vi "HTML.vi"() -> ()   [LabVIEW 2013]
uses:
  <vilib>/Utility/NIReport.llb/NI_report.lvclass
  <vilib>/Utility/NIReport.llb/Append Report Text (str wrap).vi
  <vilib>/Utility/NIReport.llb/Append Text Table to Report (wrap).vi
  <vilib>/Utility/NIReport.llb/Append Image to Report (path wrap).vi
  <vilib>/printing/OpenHTMLReport.llb/Open HTML Report in Browser (Refnum).vi
  <vilib>/Utility/NIReport.llb/NI_ReportGenerationCore.lvlib
panel:
  in  "list elements":string[](array[string])
  in  "column headers":string[](array[string])
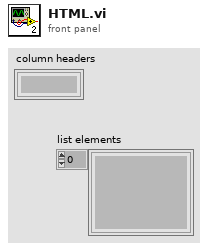
[diagram p1: front panel]
types:
  T1 = enum16{"Standard Report", "HTML", "Word", "Excel"}
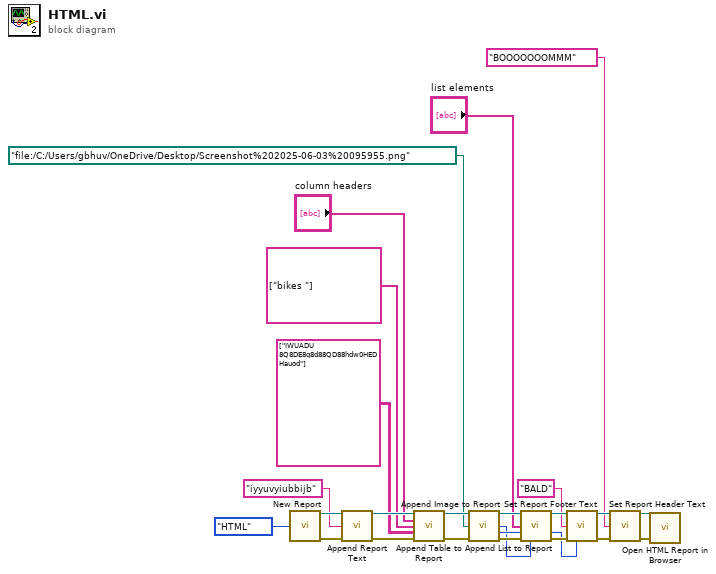
[diagram p0: block diagram]
diagram:
  n1 = call <vilib>:"New Report.vi"("report type"=T1."HTML") -> ("report out"=w25:refnum<class "NI_report.lvclass">, "error out"=w24:errorcluster)  [unwired: 13 in]
  n2 = call-poly <vilib>:"Append Report Text.vi"("report in"=w25, "text"="iyyuvyiubbijb", "error in (no error)"=w24) -> ("report out"=w22:refnum<class "NI_report.lvclass">, "error out"=w21:errorcluster)  [unwired: 9 in, 2 out]
  n3 = call-poly <vilib>:"Append Table to Report.vi"("report in"=w22, "column headers"="column headers", "row headers"=string[] ["bikes "], "text data"=string[][] [["IWUADU  8Q8DE8q8d88QD88hdw0HEDHauod"]], "error in (no error)"=w21) -> ("report out"=w18:refnum<class "NI_report.lvclass">, "error out"=w17:errorcluster)  [unwired: 7 in, 2 out]
  n4 = call-poly <vilib>:"Append Image to Report.vi"("report in"=w18, "path or URL of image"=path "file:/C:/Users/gbhuv/OneDrive/Desktop/Screenshot%202025-06-03%20095955.png", "error in (no error)"=w17) -> ("report out"=w15:refnum<class "NI_report.lvclass">, "start out (Word)"=w12:i32, "end out (Word)"=w14:i32, "error out"=w13:errorcluster)  [unwired: 9 in]
  n5 = call-dynamic "Append List to Report.vi"("report in"=w15, "list elements"="list elements", "list type (ordered)"=w14, "error in (no error)"=w13, "ordered start (1)"=w12) -> ("report out"=w9:refnum<class "NI_report.lvclass">, "end out (Word)"=w7:i32, "error out"=w8:errorcluster)  [unwired: 7 in, 1 out]
  n6 = call-dynamic "Set Report Footer Text.vi"("report in"=w9, "center footer text"="BALD", "error in (no error)"=w8, "HTML footer size"=w7) -> ("report out"=w5:refnum<class "NI_report.lvclass">, "error out"=w4:errorcluster)  [unwired: 10 in]
  n7 = call-dynamic "Set Report Header Text.vi"("report in"=w5, "center header text"="BOOOOOOOMMM", "error in (no error)"=w4) -> ("report out"=w2:refnum<class "NI_report.lvclass">, "error out"=w1:errorcluster)  [unwired: 11 in]
  n8 = call-poly <vilib>:"Open HTML Report in Browser.vi"("report in"=w2, "error in (no error)"=w1) -> ()  [unwired: 11 in, 3 out]
